vi "EventLogger.GetHandle.vi"(8 "error in":errorcluster) -> (0 "error out":errorcluster, 3 "EventLog ref":refnum<class "EventLog.lvclass">)   [LabVIEW 2019, in "Tools.lvlib"]
uses:
  Tools.lvlib
  <vilib>/NI/Event Logger Library/EventLog/EventLog.lvclass
  EventLogger.Manager.Action.ctl
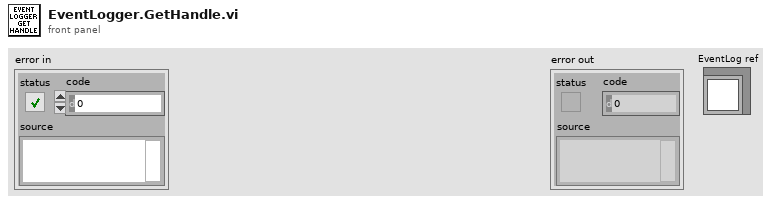
[diagram p1: front panel]
types:
  T1 = typedef "Tools.lvlib/EventLogger.Manager.Action.ctl" = enum16{"init", "get", "close"}
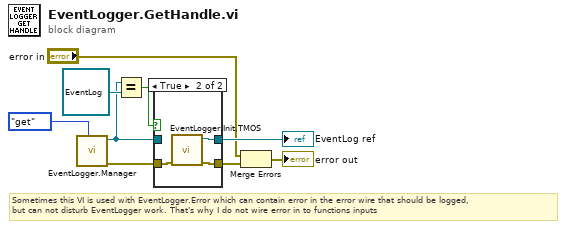
[diagram p0: block diagram]
diagram:
  # "Sometimes this VI is used with EventLogger.Error which can contain error in the error wire that should be logged, \nbut can not disturb EventLogger work. That's why I do not wire error in to functions inputs"
  n1 = call "EventLogger.Manager.vi"("action"=EventLogger.Manager.Action."get") -> ("error out"=w4:errorcluster, "EventLog ref out"=w5:refnum<class "EventLog.lvclass">)  [unwired: 9 in]
  n2 = Equal?(x=w5, y=refnum<class "EventLog.lvclass"> refnum ("EventLog ref in")) -> (x = y?=w6:bool)
  n3 = case shown="True" w6 {
    tunnel: w5 -> [w11 _]
    tunnel: w4 -> [w10 w14]
    tunnel: [w10 w13] -> w2
    tunnel: [w11 w12] -> w9
    frame False {
    }
    frame True {
      n4 = call "EventLogger.Init.TMOS.vi"("error in"=w14) -> ("error out"=w13:errorcluster, "EventLog ref out"=w12:refnum<class "EventLog.lvclass">)  [unwired: 9 in]
    }
  }
  "EventLog ref" <- w9
  n5 = Merge Errors("error in", w2) -> (→"error out":errorcluster)
